vi "客户端2.vi"() -> ()   [LabVIEW 2020]
panel:
  out "错误输出":errorcluster
  in  "停止":bool
  out "波形图":dbl[](graph)
  in  "远程端口或服务名称":u16
  in  "地址":string
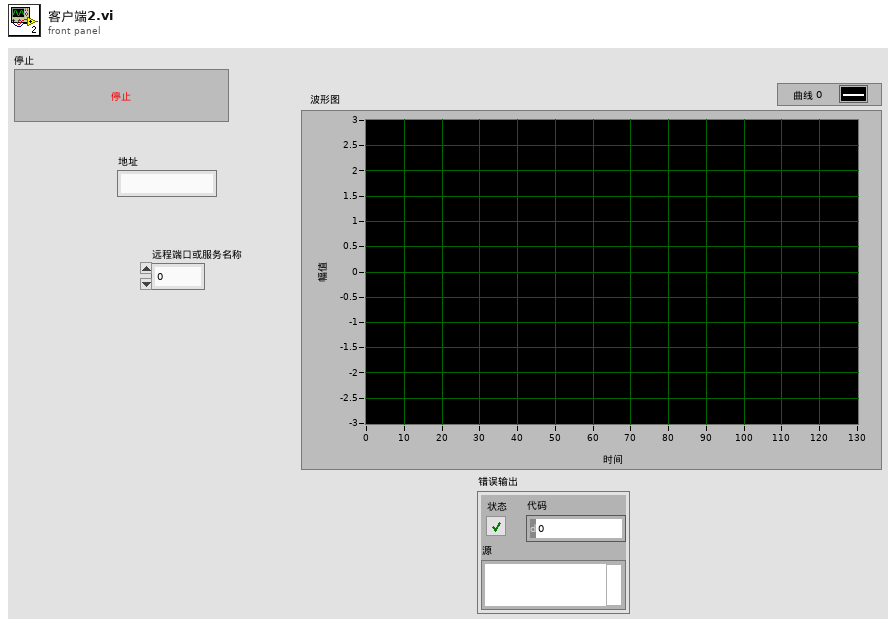
[diagram p1: front panel]
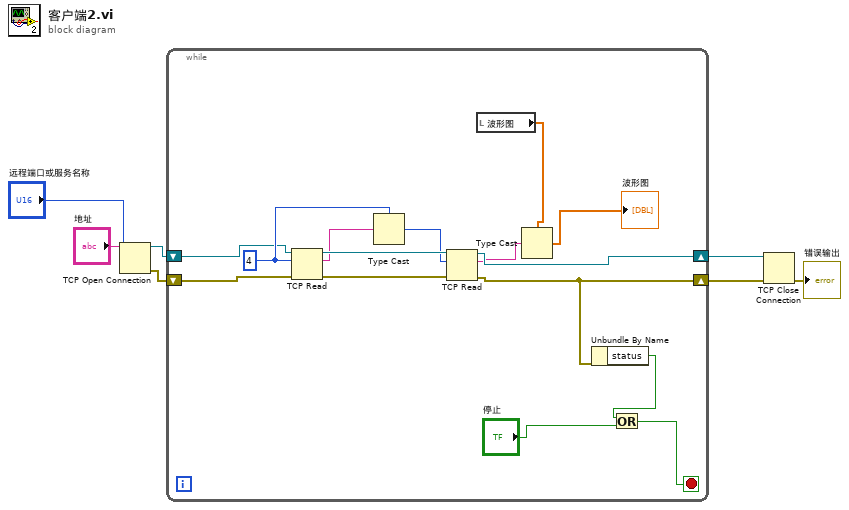
[diagram p0: block diagram]
diagram:
  n1 = TCP Open Connection(address="地址", remote port or service name="远程端口或服务名称") -> (connection ID=w5:refnum<k5>, error out=w4:errorcluster)  [unwired: 3 in]
  n2 = while {
    shift-right: [w15] -> w3
    shift-left: w5 -> [w21]
    shift-right: [w11] -> w2
    shift-left: w4 -> [w20]
    stop <- w9 stop-if-true
    w22 = 4 ("读取的字节")
    n3 = TCP Read(connection ID=w21, bytes to read=w22, error in (no error)=w20) -> (connection ID out=w19:refnum<k5>, data out=w18:string, error out=w16:errorcluster)  [unwired: 2 in]
    n4 = Type Cast(type=w22, x=w18) -> (*(type *) &x=w17:i32)
    n5 = TCP Read(connection ID=w19, bytes to read=w17, error in (no error)=w16) -> (connection ID out=w15:refnum<k5>, data out=w14:string, error out=w11:errorcluster)  [unwired: 2 in]
    n6 = local read "波形图"() -> (w12:dbl[])
    n7 = Type Cast(type=w12, x=w14) -> (*(type *) &x=→"波形图":dbl[])
    n8 = Unbundle By Name(w11) -> ("status"=w10:bool)
    n9 = Or(x=w10, y="停止") -> (x .or. y?=w9:bool)
  }
  n10 = TCP Close Connection(connection ID=w3, error in (no error)=w2) -> (error out=→"错误输出":errorcluster)  [unwired: 1 in, 1 out]
